vi "Actor Core.vi"(8 "error in":errorcluster, 11 "Generador in":refnum<class "Generador.lvclass">) -> (0 "error out":errorcluster, 3 "Actor out":refnum<class "Actor.lvclass">)   [LabVIEW 2020, in "Generador.lvlib" / "Generador.lvclass"]
doc: "(<B>Filename</B>: Actor Framework.lvlib:Actor.lvclass:Actor Core.vi)\n\nReceives messages to the actor, reacts to them, and initiates any error handling that may shut the actor down.\n\nDescendant classes may override this VI to append parallel tasks for the actor to complete while it handles messages. Overrides use the Call Parent Class Method node."
uses:
  Generador.lvclass
  <vilib>/ActorFramework/Actor/Actor.lvclass
  <vilib>/ActorFramework/Stop Msg/Stop Msg.lvclass
  C:/Program Files (x86)/National Instruments/LabVIEW 2020/vi.lib/ActorFramework/Actor/Actor.lvclass
  C:/Users/Pablo/Actor_Framework-02/Actor_Framework-02/Generador/Generador/Generador.lvclass
panel:
  in  "Stop":bool
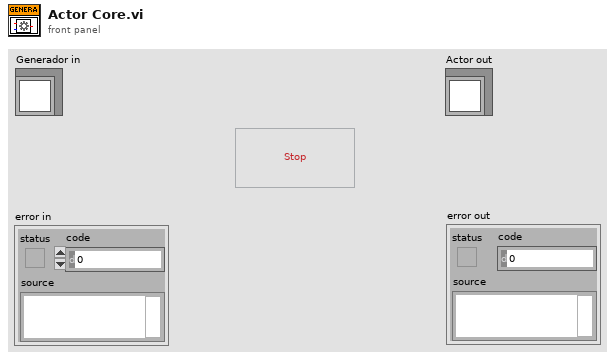
[diagram p1: front panel]
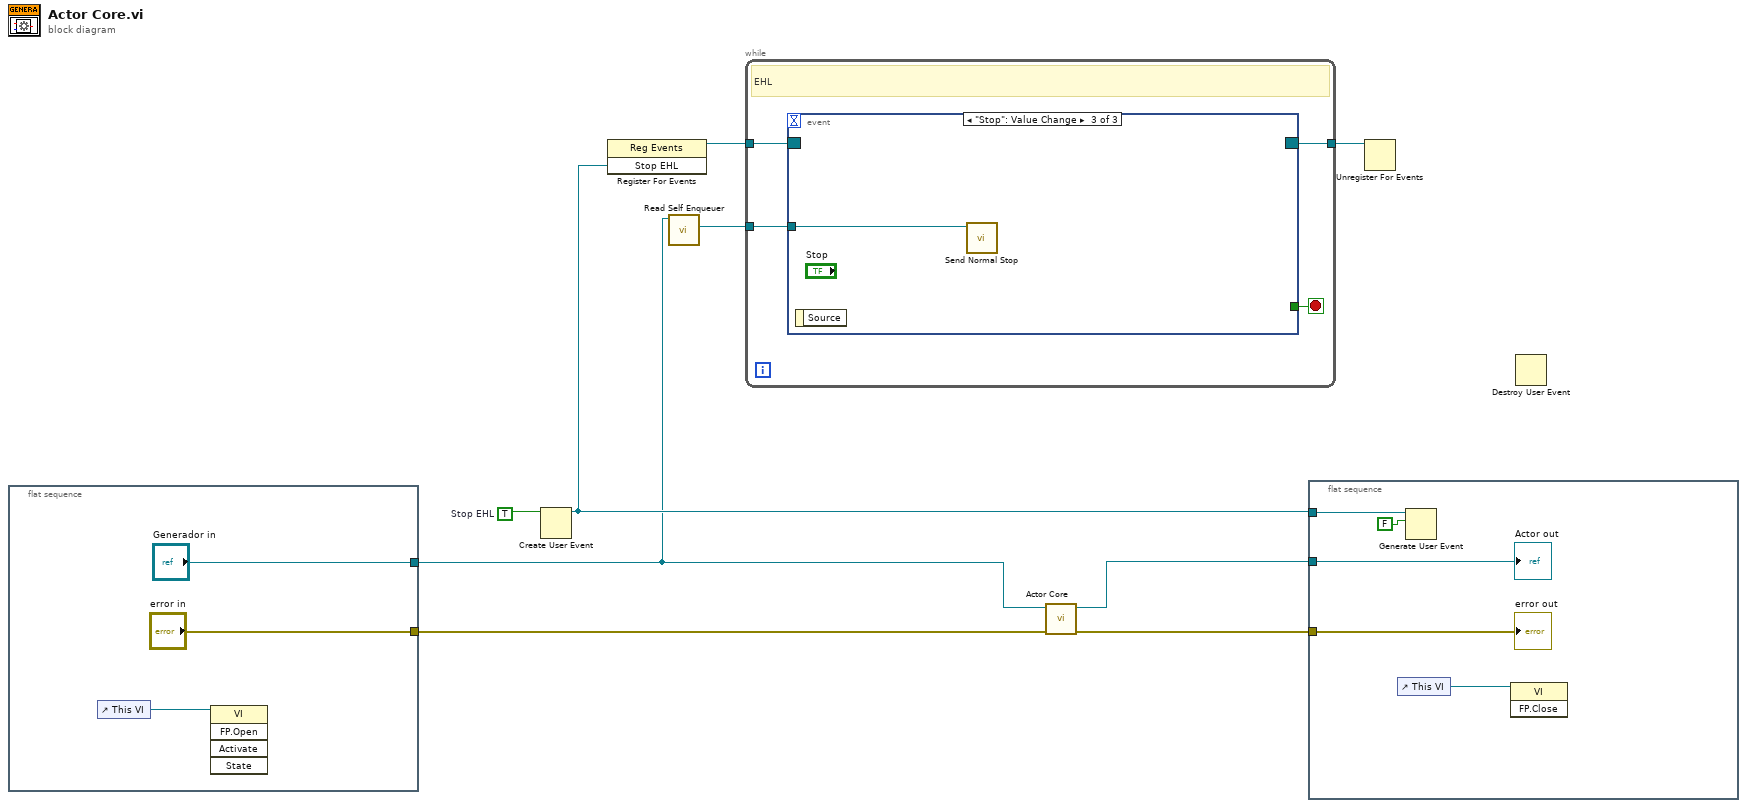
[diagram p0: block diagram]
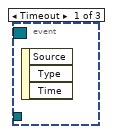
[diagram p2: hidden frame]
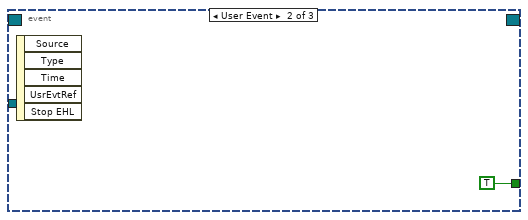
[diagram p3: hidden frame]
diagram:
  w5 = TRUE  # Stop EHL
  n1 = flat-sequence {
    tunnel: ["error in"] -> w7
    tunnel: ["Generador in"] -> w1
    frame #0 {
      n2 = control-ref of="This VI"() -> (w10:refnum<vi>)
      n3 = invoke class="VI" method="FP.Open"(reference=w10) -> ()  [unwired: 4 in, 5 out]
    }
  }
  n4 = Create User Event(user event datatype=w5) -> (user event=w3:refnum<user-event>)  [unwired: 1 in, 1 out]
  n5 = register-events(w3) -> (reference out=w6:refnum<event-registration>)  [unwired: 2 in, 1 out]
  n6 = call <vilib>:"Read Self Enqueuer.vi"("Actor"=w1) -> ("Self Enqueuer"=w2:refnum<class "Message Enqueuer.lvclass">)  [unwired: 10 in]
  n7 = while {
    tunnel: w6 -> [w16]
    tunnel: [w15] -> w4
    tunnel: w2 -> [w13]
    stop <- w14 stop-if-true
    # "EHL"
    n8 = event shown="[2] \"Stop\": Value Change" {
      selector: w16 -> [_ _ _]
      dyn-events: [_ _ _] -> w15
      timeout: _ -> [_ _ _]
      tunnel: [_ TRUE _] -> w14
      tunnel: w13 -> [_ _ w18]
      event Timeout {
        n9 = event-data() -> ()  [unwired: 1 in, 3 out]
      }
      event User Event {
        n10 = event-data() -> ()  [unwired: 1 in, 5 out]
      }
      event "Stop": Value Change {
        n11 = event-data() -> ()  [unwired: 1 in, 1 out]
        n12 = call <vilib>:"Send Normal Stop.vi"("Message Enqueuer"=w18) -> ()  [unwired: 10 in, 1 out]
      }
    }
  }
  n13 = call-parent "Actor Core.vi"("error in"=w7, "Actor in"=w1) -> ("error out"=w9:errorcluster, "Actor out"=w8:refnum<class "Actor.lvclass">)  [unwired: 8 in]
  n14 = flat-sequence {
    tunnel: w9 -> [w23]
    tunnel: w8 -> [w22]
    tunnel: w3 -> [w20]
    frame #0 {
      n15 = control-ref of="This VI"() -> (w21:refnum<vi>)
      n16 = Generate User Event(user event=w20, event data cluster=FALSE ("event data")) -> ()  [unwired: 2 in, 2 out]
      n17 = invoke class="VI" method="FP.Close"(reference=w21) -> ()  [unwired: 2 in, 3 out]
      "error out" <- w23
      "Actor out" <- w22
    }
  }
  n18 = Unregister For Events(event registration refnum=w4) -> ()  [unwired: 1 in, 1 out]
  n19 = Destroy User Event() -> ()  [unwired: 2 in, 1 out]
